vi "Assert Log File Size.vi"(8 "error in":errorcluster, 9 "Expected size of file in bytes":i64, 10 "file path":path, 11 "Embedded Data Logger System Tests in":refnum<class "Embedded Data Logger Windows System Tests.lvclass">) -> (0 "error out":errorcluster, 3 "Embedded Data Logger System Tests out":refnum<class "Embedded Data Logger Windows System Tests.lvclass">)   [LabVIEW 2027, in "Embedded Data Logger Windows System Tests.lvclass"]
uses:
  Embedded Data Logger Windows System Tests.lvclass
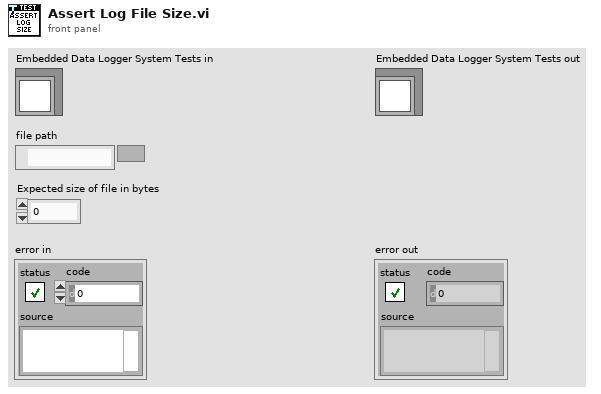
[diagram p1: front panel]
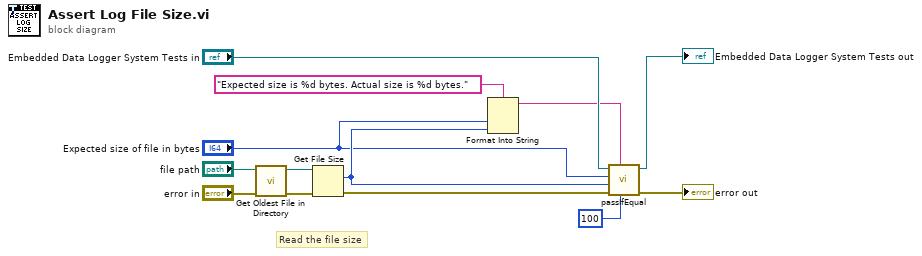
[diagram p0: block diagram]
diagram:
  # "Read the file size"
  n1 = call "Get Oldest File in Directory.vi"("error in"="error in", "Directory"="file path") -> ("error out"=w6:errorcluster, "Oldest File"=w4:path)  [unwired: 8 in]
  n2 = Get File Size(file=w4, error in=w6) -> (size (in bytes)=w3:i64, 0:w8:errorcluster)  [unwired: 1 out]
  n3 = Format Into String(format string="Expected size is %d bytes. Actual size is %d bytes.", "Expected size of file in bytes", w3) -> (resulting string=w10:string)  [unwired: 2 in, 1 out]
  n4 = call-dynamic "passIfEqual.vi"("delta (optional)"=i64 100 ("size (in bytes)"), "custom report message (\"\")"=w10, "error in (no error)"=w8, "y"=w3, "x"="Expected size of file in bytes", "TestCase in"="Embedded Data Logger System Tests in") -> ("error out"=→"error out":errorcluster, "TestCase out"=→"Embedded Data Logger System Tests out":refnum<class "Embedded Data Logger Windows System Tests.lvclass">)  [unwired: 4 in]
